vi "Refresh Throttle Listbox.vi"(8 "Data":T1(array[cluster]), 11 "Throttle Data":refnum<vi>) -> ()   [LabVIEW 2016]
uses:
  <vilib>/Utility/miscctls.llb/LVRowAndColumnTypeDef.ctl
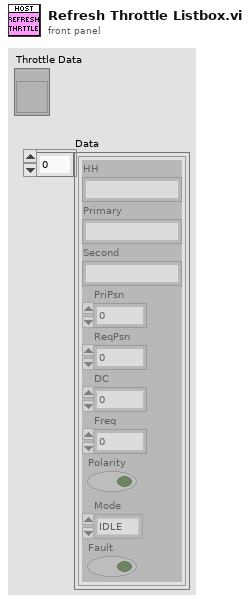
[diagram p1: front panel]
types:
  T1 = cluster{"HH":string, "Primary":string, "Second":string, "PriPsn":sgl, "ReqPsn":sgl, "DC":sgl, "Freq":sgl, "Polarity":bool, "Mode":enum16{"IDLE", "POSITION CALIBRATION", "CONTROL CALIBRATION", "CONTROL"}, "Fault":bool}[]
  T2 = typedef "LVRowAndColumnTypeDef.ctl" = cluster{"Row":i32, "Column":i32}
  T3 = enum16{"IDLE", "POSITION CALIBRATION", "CONTROL CALIBRATION", "CONTROL"}
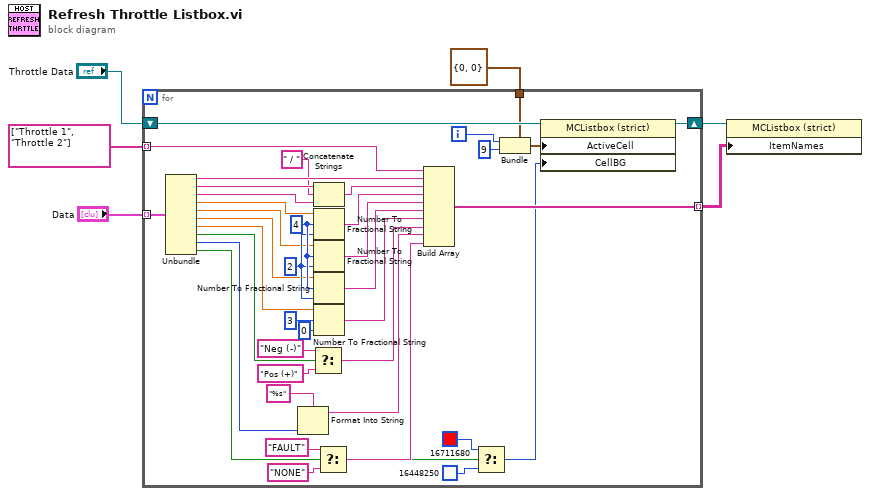
[diagram p0: block diagram]
diagram:
  n1 = for {
    tunnel: "Data" -> [w46] mode=indexing
    tunnel: [w44] -> w6 mode=indexing
    tunnel: string[] ["Throttle 1", "Throttle 2"] -> [w40] mode=indexing
    shift-right: [w15] -> w2
    shift-left: "Throttle Data" -> [w16]
    tunnel: T2 {"Row"=0, "Column"=0} ("Active Cell:Active Cell") -> [w13]
    i -> [w11]
    w42 = i16 2 ("precision (6)")
    w43 = i16 4 ("width (-)")
    n2 = Unbundle(w46) -> ("HH"=w45:string, "Primary"=w37:string, "Second"=w38:string, "PriPsn"=w35:sgl, "ReqPsn"=w34:sgl, "DC"=w33:sgl, "Freq"=w32:sgl, "Polarity"=w26:bool, "Mode"=w22:T3, "Fault"=w10:bool)
    n3 = Format Into String(format string="%s", w22) -> (resulting string=w20:string)  [unwired: 2 in, 1 out]
    n4 = Select(t="Neg (-)" ("F-format string"), s=w26, f="Pos (+)" ("F-format string")) -> (s? t:f=w25:string)
    n5 = Concatenate Strings(w37, " / " ("string"), w38) -> (w39:string)
    n6 = Number To Fractional String(number=w35, width (-)=w43, precision (6)=w42) -> (F-format string=w31:string)  [unwired: 1 in]
    n7 = Number To Fractional String(number=w34, width (-)=w43, precision (6)=w42) -> (F-format string=w30:string)  [unwired: 1 in]
    n8 = Number To Fractional String(number=w33, width (-)=w43, precision (6)=w42) -> (F-format string=w29:string)  [unwired: 1 in]
    n9 = Number To Fractional String(number=w32, width (-)=i16 3, precision (6)=i16 0) -> (F-format string=w28:string)  [unwired: 1 in]
    n10 = Select(t="FAULT" ("F-format string"), s=w10, f="NONE" ("F-format string")) -> (s? t:f=w18:string)
    n11 = Build Array(w40, w45, w39, w31, w30, w29, w28, w25, w20, w18) -> (w44:string[])
    n12 = Select(t=u32 16711680, s=w10, f=u32 16448250) -> (s? t:f=w9:u32)
    n13 = Bundle(cluster=w13, "Row"=w11, "Column"=9) -> (w14:T2)
    n14 = property class="MCListbox (strict)"(reference=w16, "ActiveCell"=w14, "CellBG"=w9) -> (reference out=w15:refnum<vi>)  [unwired: 1 in, 1 out]
  }
  n15 = property class="MCListbox (strict)"(reference=w2, "ItemNames"=w6) -> ()  [unwired: 1 in, 2 out]
